vi "2 NoSailGoodness.vi"(10 "Heading to Test":dbl) -> (2 "Goodness":dbl)   [LabVIEW 2011]
uses:
  2 Classes/Waypoint/Waypoint.lvclass
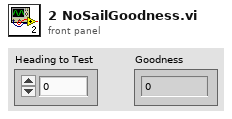
[diagram p1: front panel]
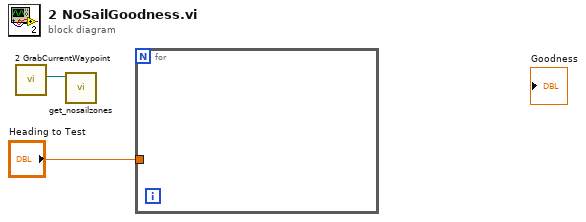
[diagram p0: block diagram]
diagram:
  n1 = call "2 GrabCurrentWaypoint.vi"() -> ("Current Waypoint"=w1:refnum<class "Waypoint.lvclass">)  [unwired: 11 in]
  n2 = call-dynamic "get_nosailzones.vi"("Waypoint in"=w1) -> ()  [unwired: 9 in, 2 out]
  n3 = for {
    tunnel: "Heading to Test" -> [_]
  }
